vi "Close FP.vi"(8 "Error In":errorcluster, 11 "VI Ref":refnum<vi>) -> (0 "Error Out":errorcluster)   [LabVIEW 2014, in "LMH-Toolbox.lvlib"]
doc: "Close the VI front panel. If the user is holding shift while the FP would close it is left open (for debugging)."
uses:
  <vilib>/MakerHub/Toolbox/LMH-Toolbox.lvlib
  <vilib>/Utility/inputDevices.llb/keyboardAcquire.vi
  <vilib>/Utility/inputDevices.llb/closeKeyboard.vi
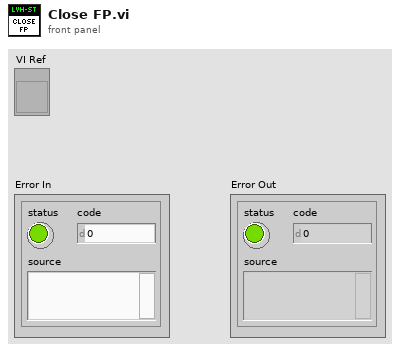
[diagram p1: front panel]
types:
  T1 = enum16{"0", "1", "2", "3", "4", "5", "6", "7", "8", "9", "A", "B", "C", "D", "E", "F", "G", "H", "I", "J", "K", "L", "M", "N", "O", "P", "Q", "R", "S", "T", "U", "V", "W", "X", "Y", "Z", "F1", "F2", "F3", "F4", "F5", "F6", "F7", "F8", "F9", "F10", "F11", "F12", "F13", "F14", "F15", "ADD", "BACK", "BACKSLASH", "CAPITAL", "COMMA", "DECIMAL", "DELETE", "DIVIDE", "DOWN", "END", "EQUALS", "ESCAPE", "GRAVE (`)", "HOME", "INSERT", "LBRACKET", "LCONTROL", "LEFT", "L ALT", "LSHIFT", "LWIN", "MINUS", "MULTIPLY", "NEXT", "NUMLOCK", "NUMPAD_0", "NUMPAD_1", "NUMPAD_2", "NUMPAD_3", "NUMPAD_4", "NUMPAD_5", "NUMPAD_6", "NUMPAD_7", "NUMPAD_8", "NUMPAD_9", "PAUSE", "PERIOD", "PRIOR (PG UP)", "RBRACKET", "RCONTROL", "RETURN", "RIGHT", "R ALT", "RSHIFT", "RWIN", "SCROLL", "SEMICOLON", "SLASH", "SPACE", "SUBTRACT", "TAB", "UP", "ENTER (num pad)", "' (quote)"}[]
  T2 = enum16{"0", "1", "2", "3", "4", "5", "6", "7", "8", "9", "A", "B", "C", "D", "E", "F", "G", "H", "I", "J", "K", "L", "M", "N", "O", "P", "Q", "R", "S", "T", "U", "V", "W", "X", "Y", "Z", "F1", "F2", "F3", "F4", "F5", "F6", "F7", "F8", "F9", "F10", "F11", "F12", "F13", "F14", "F15", "ADD", "BACK", "BACKSLASH", "CAPITAL", "COMMA", "DECIMAL", "DELETE", "DIVIDE", "DOWN", "END", "EQUALS", "ESCAPE", "GRAVE (`)", "HOME", "INSERT", "LBRACKET", "LCONTROL", "LEFT", "L ALT", "LSHIFT", "LWIN", "MINUS", "MULTIPLY", "NEXT", "NUMLOCK", "NUMPAD_0", "NUMPAD_1", "NUMPAD_2", "NUMPAD_3", "NUMPAD_4", "NUMPAD_5", "NUMPAD_6", "NUMPAD_7", "NUMPAD_8", "NUMPAD_9", "PAUSE", "PERIOD", "PRIOR (PG UP)", "RBRACKET", "RCONTROL", "RETURN", "RIGHT", "R ALT", "RSHIFT", "RWIN", "SCROLL", "SEMICOLON", "SLASH", "SPACE", "SUBTRACT", "TAB", "UP", "ENTER (num pad)", "' (quote)"}
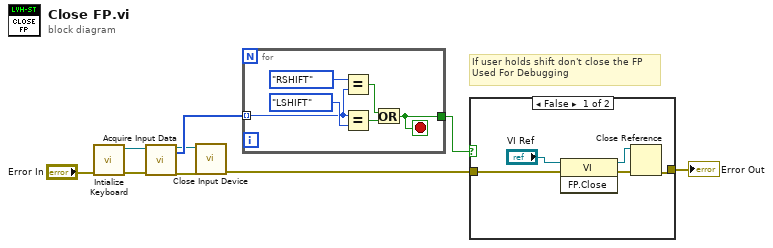
[diagram p0: block diagram]
diagram:
  # "If user holds shift don't close the FP\nUsed For Debugging"
  n1 = call <vilib>:"Intialize Keyboard.vi"("error in (no error)"="Error In") -> ("error out"=w4:errorcluster, "device ID"=w5:refnum<k1>)  [unwired: 9 in]
  n2 = call-poly <vilib>:"Acquire Input Data.vi"("device ID"=w5, "error in (no error)"=w4) -> ("device ID"=w7:refnum<k1>, "keys pressed"=w8:T1, "error out"=w6:errorcluster)  [unwired: 15 in]
  n3 = call-poly <vilib>:"Close Input Device.vi"("error in (no error)"=w6, "device ID"=w7) -> ("error out"=w3:errorcluster)  [unwired: 8 in]
  n4 = for {
    tunnel: w8 -> [w12] mode=indexing
    tunnel: [w10] -> w2
    stop <- w10 stop-if-true
    n5 = Equal?(x=T2."RSHIFT", y=w12) -> (x = y?=w14:bool)
    n6 = Equal?(x=w12, y=T2."LSHIFT" ("x")) -> (x = y?=w11:bool)
    n7 = Or(x=w14, y=w11) -> (x .or. y?=w10:bool)
  }
  n8 = case shown="False" w2 {
    tunnel: [w20 w21] -> w9
    tunnel: w3 -> [w17 w21]
    frame False {
      n9 = invoke class="VI" method="FP.Close"(reference="VI Ref", error in=w17) -> (reference out=w18:refnum<vi>, error out=w19:errorcluster)  [unwired: 1 in, 1 out]
      n10 = Close Reference(reference=w18, error in (no error)=w19) -> (error out=w20:errorcluster)
    }
    frame True {
    }
  }
  "Error Out" <- w9
